vi "WSP2_InsertProcessDataWithFails.vi"(4 "Employee":string, 5 "FailString":string, 6 "EndTime":string, 7 "EntryTime":string, 8 "PassFail":i32, 9 "ProcessName":string, 10 "StationName":string, 11 "SerialNumber":string) -> (2 "ReplyTrace":string)   [LabVIEW 2017]
uses:
  C:/ClubCar EOL/WSConnector/WSConnector.dll
  WSConnector/WSConnector.dll
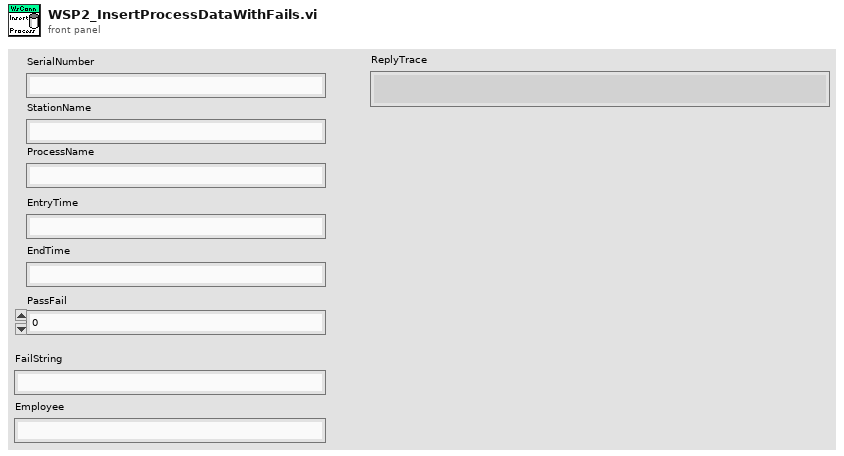
[diagram p1: front panel]
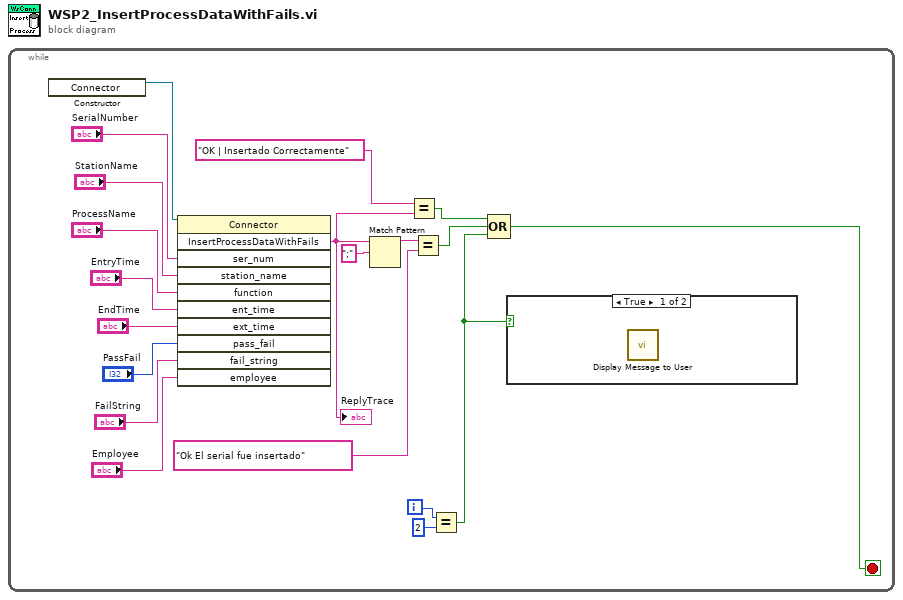
[diagram p0: block diagram]
diagram:
  n1 = while {
    i -> [w4]
    stop <- w2 stop-if-true
    n2 = constructor class="Connector"() -> (reference out=w12:refnum<k24>)  [unwired: 3 in, 2 out]
    n3 = invoke class="Connector" method="InsertProcessDataWithFails"(reference=w12, "ser_num"="SerialNumber", "station_name"="StationName", "function"="ProcessName", "ent_time"="EntryTime", "ext_time"="EndTime", "pass_fail"="PassFail", "fail_string"="FailString", "employee"="Employee") -> ("InsertProcessDataWithFails"=w6:string)  [unwired: 2 in, 10 out]
    "ReplyTrace" <- w6
    n4 = Match Pattern(string=w6, regular expression=";") -> (before substring=w9:string)  [unwired: 1 in, 3 out]
    n5 = Equal?(x="OK | Insertado Correctamente", y=w6) -> (x = y?=w7:bool)
    n6 = Equal?(x=w9, y="Ok El serial fue insertado") -> (x = y?=w8:bool)
    n7 = Equal?(x=w4, y=2) -> (x = y?=w1:bool)
    n8 = Compound Arithmetic op=OR(w7, w8, w1) -> (w2:bool)
    n9 = case shown="True" w1 {
      frame True {
        n10 = call "Display Message to User"() -> ()  [unwired: 10 in, 2 out]
      }
      frame False {
      }
    }
  }
